vi "Set Voltage.vi"(8 "errorIN":errorcluster caption="Error", 9 "milliseconds to wait (0)":u32, 10 "Voltage in":dbl, 11 "LCD in":refnum<class "LCD Retarder.lvclass">) -> (0 "errorOUT":errorcluster caption="Error out", 2 "Retardance out":dbl[unit], 3 "LCD out":refnum<class "LCD Retarder.lvclass">)   [LabVIEW 2017, in "LCD Retarder.lvclass"]
uses:
  LCD Retarder.lvclass
  LCD Retarder.lvclass/LCD Retarder.ctl
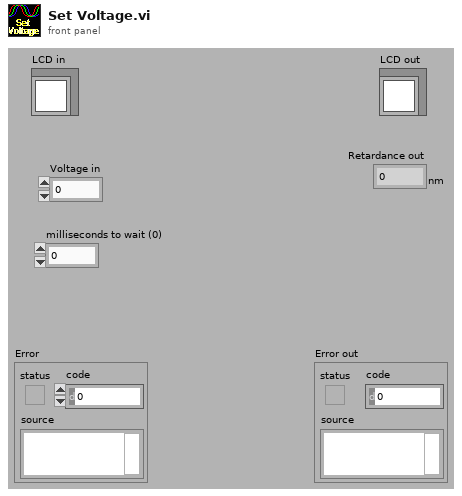
[diagram p1: front panel]
types:
  T1 = cluster{"Device Handle":u32, "Pipe 0 Handle":u32, "Pipe 1 Handle":u32}
  T2 = typedef "Readable.lvclass/X array.ctl" = T3[]
  T3 = typedef "Readable.lvclass/X.ctl" = dbl
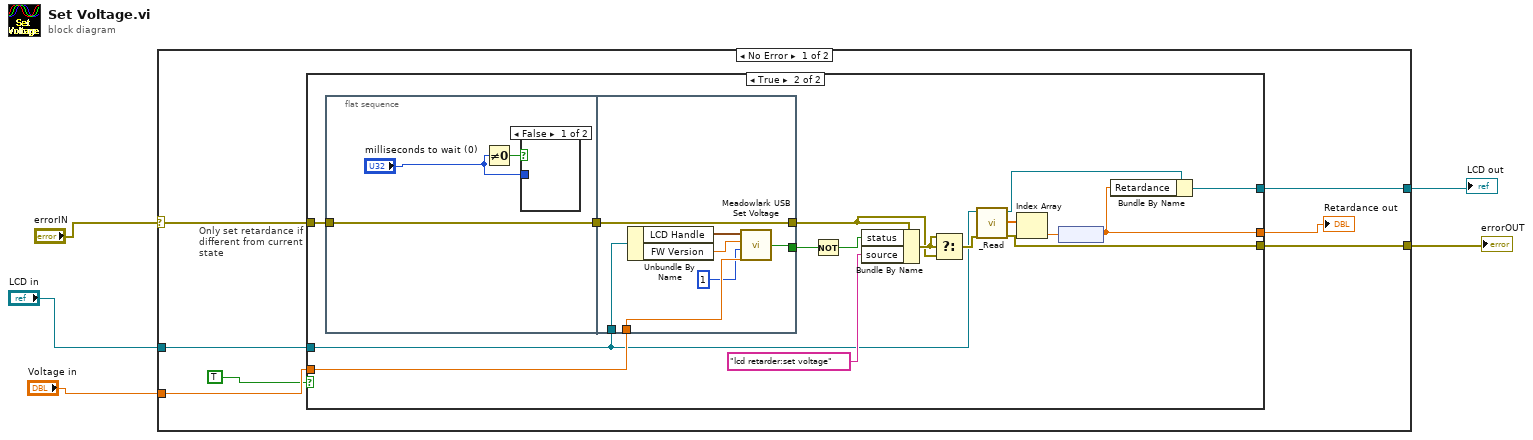
[diagram p0: block diagram]
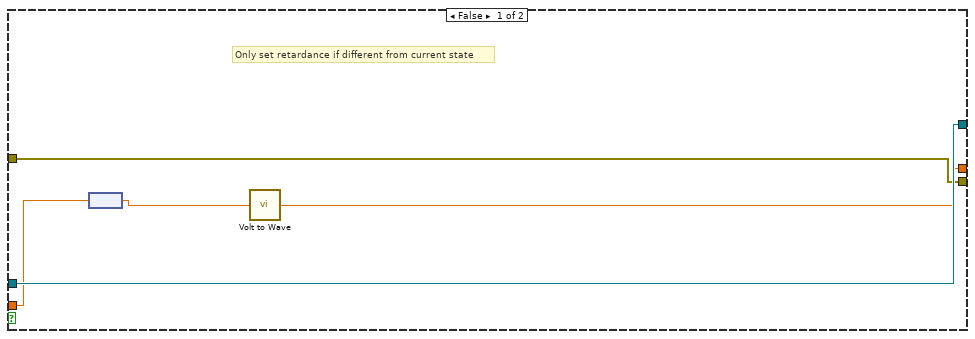
[diagram p2: hidden frame]
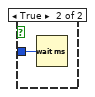
[diagram p3: hidden frame]
diagram:
  n1 = case shown="No Error" "errorIN" {
    selector: "errorIN" -> [w11 w45]
    tunnel: "Voltage in" -> [w8 _]
    tunnel: "LCD in" -> [w9 w46]
    tunnel: [w10 w46] -> w1
    tunnel: [w12 w45] -> w2
    frame No Error {
      n2 = case "Only set retardance if different from current state" shown="True" TRUE {
        tunnel: [w16 w20] -> w12
        tunnel: w11 -> [w16 w28]
        tunnel: [w17 w26] -> w10
        tunnel: w8 -> [w15 w23]
        tunnel: w9 -> [w17 w18]
        tunnel: [w13 w24] -> w6
        frame False {
          # "Only set retardance if different from current state"
          n3 = node(w15) -> (w14:dbl[unit])
          n4 = call "Volt to Wave.vi"("Voltage"=w14) -> ("Retardance"=w13:dbl[unit])
        }
        frame True {
          n5 = flat-sequence {
            tunnel: w28 -> [w36]
            tunnel: [w36] -> w33
            tunnel: [w44] -> w29
            tunnel: w33 -> [w44]
            tunnel: w18 -> [w43]
            tunnel: w23 -> [w42]
            tunnel: [w38] -> w27
            frame #0 {
              n6 = Not Equal To 0?(x="milliseconds to wait (0)") -> (x != 0?=w35:bool)
              n7 = case shown="False" w35 {
                tunnel: "milliseconds to wait (0)" -> [_ w37]
                frame False {
                }
                frame True {
                  n8 = Wait (ms)(milliseconds to wait=w37) -> ()  [unwired: 1 out]
                }
              }
            }
            frame #1 {
              n9 = Unbundle By Name(w43) -> ("LCD Handle"=w39:T1, "FW Version"=w40:dbl)
              n10 = call "Meadowlark USB Set Voltage.VI"("LC Voltage"=w42, "LC Channel"=1, "FW Version"=w40, "USB Open Device Cluster"=w39) -> ("Successful?"=w38:bool)
            }
          }
          n11 = Not(x=w27) -> (.not. x?=w32:bool)
          n12 = Bundle By Name(cluster=w29, "status"=w32, "source"="lcd retarder:set voltage") -> (w31:errorcluster)
          n13 = Select(t=w31, s=w31, f=w29) -> (s? t:f=w19:errorcluster)
          n14 = call-dynamic "_Read.vi"("errorIN"=w19, "LCD in"=w18) -> ("errorOUT"=w20:errorcluster, "X array"=w21:T2, "LCD out"=w22:refnum<class "LCD Retarder.lvclass">)  [unwired: 7 in]
          n15 = Index Array(array=w21) -> (element=w25:T3)  [unwired: 1 in]
          n16 = node(w25) -> (w24:dbl[unit])
          n17 = Bundle By Name(cluster=w22, "Retardance"=w24) -> (w26:refnum<class "LCD Retarder.lvclass">)
        }
      }
      "Retardance out" <- w6
    }
    frame Error {
    }
  }
  "errorOUT" <- w2
  "LCD out" <- w1
